vi "set_storage_mode.vi"(8 "error in (no error)":errorcluster, 10 "type":T1, 11 "ImageCollection.lvclass in":refnum<class "ImageCollection.lvclass">) -> (0 "error out":errorcluster, 3 "ImageCollection.lvclass out":refnum<class "ImageCollection.lvclass">)   [LabVIEW 2010, in "ImageCollection.lvclass"]
uses:
  ImageCollection.lvclass
  storage_mode_enum.ctl
  ImageCollection.lvclass/ImageCollection.ctl
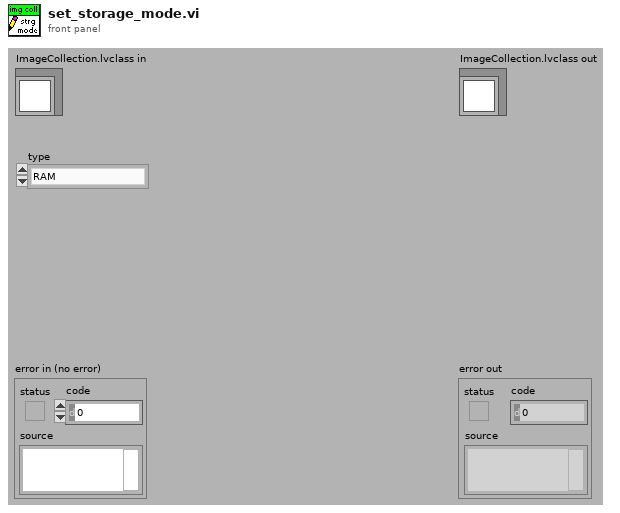
[diagram p1: front panel]
types:
  T1 = typedef "ImageCollection.lvclass/storage_mode_enum.ctl" = enum16{"RAM", "single files", "multipage TIFF (read-only)"}
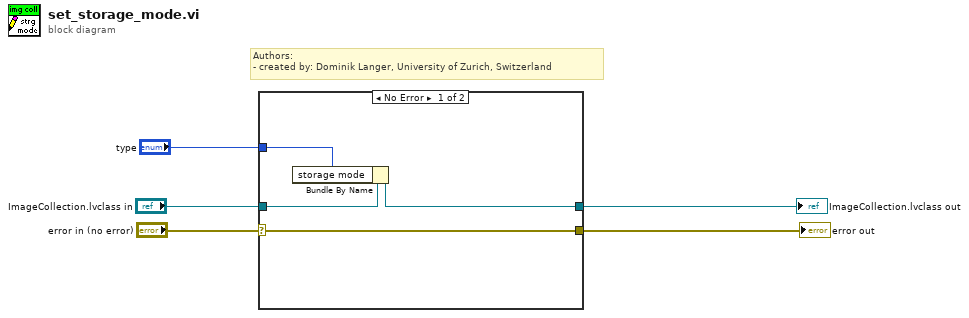
[diagram p0: block diagram]
diagram:
  # "Authors: \n- created by: Dominik Langer, University of Zurich, Switzerland"
  n1 = case shown="No Error" "error in (no error)" {
    selector: "error in (no error)" -> [w7 w10]
    tunnel: [w7 w10] -> w4
    tunnel: [w6 w11] -> w2
    tunnel: "ImageCollection.lvclass in" -> [w9 w11]
    tunnel: "type" -> [w8 _]
    frame No Error {
      n2 = Bundle By Name(cluster=w9, "storage mode"=w8) -> (w6:refnum<class "ImageCollection.lvclass">)
    }
    frame Error {
    }
  }
  "error out" <- w4
  "ImageCollection.lvclass out" <- w2
